vi "API PUT Attachments.vi"(8 "error in (no error)":errorcluster, 9 "Buffer":string, 10 "API Token":string="apitoken 2096a662-4947-42f5-97bc-84cfdf20fe4e:bc240510-8f48-43e3-889a-471659905c2e", 11 "API Endpoint Url":string="https://api.dev.enlil.io/api/v1/document_revisions/external/ALI00017/draft") -> (0 "error out":errorcluster, 4 "Response body":string, 5 "Responce headers":string)   [LabVIEW 2017]
uses:
  <vilib>/httpClient/PUTBuffer.vi
  <vilib>/httpClient/LabVIEWHTTPClient.lvlib
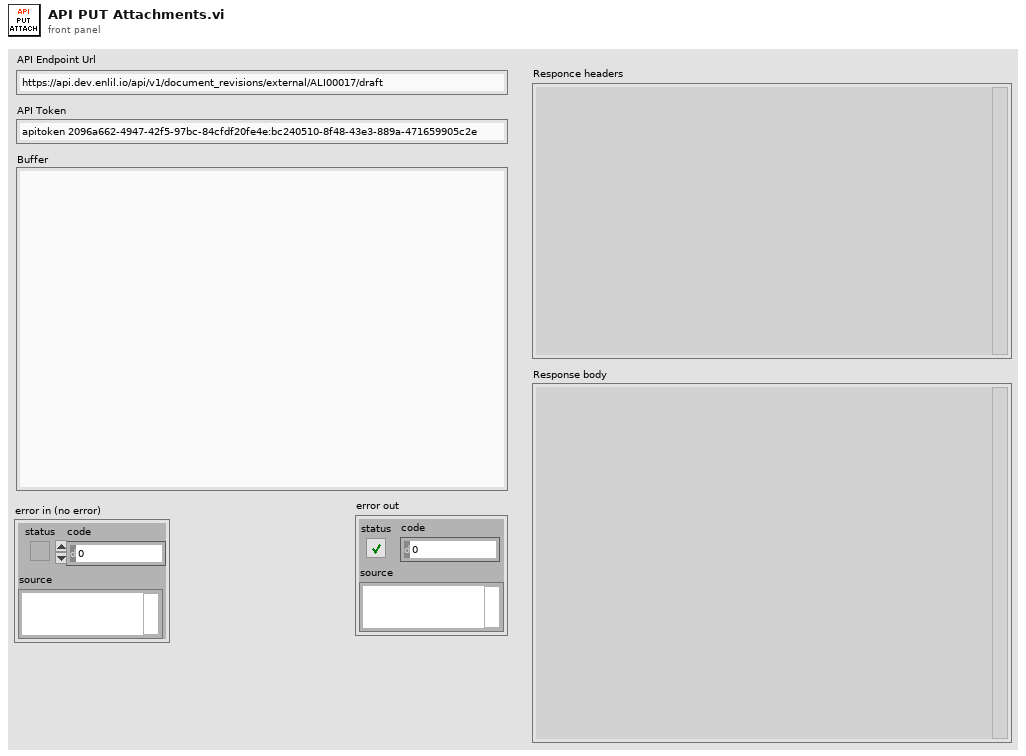
[diagram p1: front panel]
types:
  T1 = typedef "LabVIEWHTTPClient.lvlib/ClientHandle.ctl" = refnum<k1>
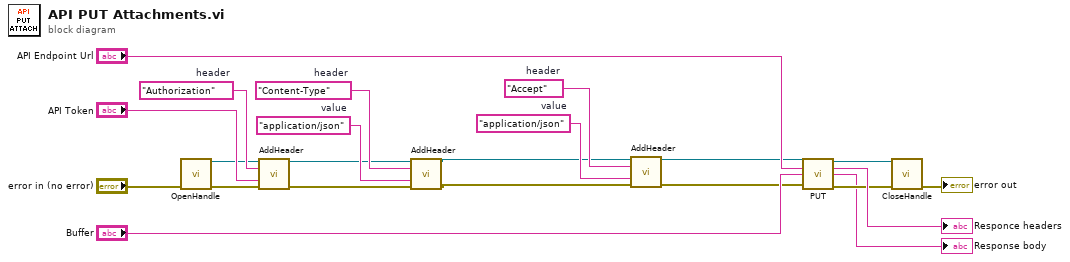
[diagram p0: block diagram]
diagram:
  w5 = "application/json"  # value
  w6 = "Accept"  # header
  w20 = "application/json"  # value
  w19 = "Content-Type"  # header
  w22 = "Authorization"  # header
  n1 = call <vilib>:"OpenHandle.vi"("error in (no error)"="error in (no error)") -> ("client handle out"=w9:T1, "error out"=w12:errorcluster)  [unwired: 13 in]
  n2 = call <vilib>:"AddHeader.vi"("client handle"=w9, "header"=w22, "value"="API Token", "error in (no error)"=w12) -> ("client handle out"=w10:T1, "error out"=w11:errorcluster)  [unwired: 10 in]
  n3 = call <vilib>:"AddHeader.vi"("client handle"=w10, "header"=w19, "value"=w20, "error in (no error)"=w11) -> ("client handle out"=w3:T1, "error out"=w4:errorcluster)  [unwired: 10 in]
  n4 = call <vilib>:"AddHeader.vi"("client handle"=w3, "header"=w6, "value"=w5, "error in (no error)"=w4) -> ("client handle out"=w2:T1, "error out"=w1:errorcluster)  [unwired: 10 in]
  n5 = call-poly <vilib>:"PUT.vi"("client handle"=w2, "url"="API Endpoint Url", "buffer"="Buffer", "error in (no error)"=w1) -> ("client handle out"=w14:T1, "headers"=→"Responce headers":string, "body"=→"Response body":string, "error out"=w15:errorcluster)  [unwired: 8 in]
  n6 = call <vilib>:"CloseHandle.vi"("client handle"=w14, "error in (no error)"=w15) -> ("error out"=→"error out":errorcluster)  [unwired: 13 in]
